vi "Reason List.vi"(8 "error in (no error)":errorcluster, 11 "Ref In":T1={"MS SQL Connection"=refnum, "UDL File"=path "", "Time"="", "DCODE"="", "WIP+1"=0, "MC No?"=0, "POKAYOKE?"=FALSE, "Expected Result"="", "Result [Status]"="", "Clock"=0.0, "RFID"="", "WIP Queue"=refnum, "TS Parameter"={"ProfitCenterCode"="", "LineCode"="", "WorkOrderNumber"="", "Model"="", "Model_with_Prefix"="", "VendorCode"="", "SetParameterDateCode"="", "PokaYoke"=0, "Target"=1, "Live_DateCode"="", "CustomerPartNumber"="", "Hand"="", "sBarcode"=FALSE, "FCA"=0, "Ent_Stamp"=timestamp(0 s since 1904-01-01), "STS_CD"=0.0}, "Data_Queue"=[], "RFID Serial No."=""} {"TS Parameter"."FCA" format="%01d"; "TS Parameter"."Target" min=1 max=100000; "TS Parameter"."PokaYoke" min=0 max=1}) -> (0 "error out":errorcluster)   [LabVIEW 2020]
uses:
  Controls/Loss_type.ctl
  Controls/TD SQL.ctl
  <vilib>/addons/database/Connection.llb/Conn ObjectReference.ctl
  Controls/WIP_State.ctl
  Controls/TS_Parameter.ctl
  <vilib>/addons/database/NI_Database_API.lvlib
panel:
  in  "Refresh":bool
  in  "Exit":bool
  in  "Del":bool
  in  "Change":bool
  in  "Add":bool
  in  "Reason":string
  in  "Code":i32(listbox)
  in  "Code Type":T4
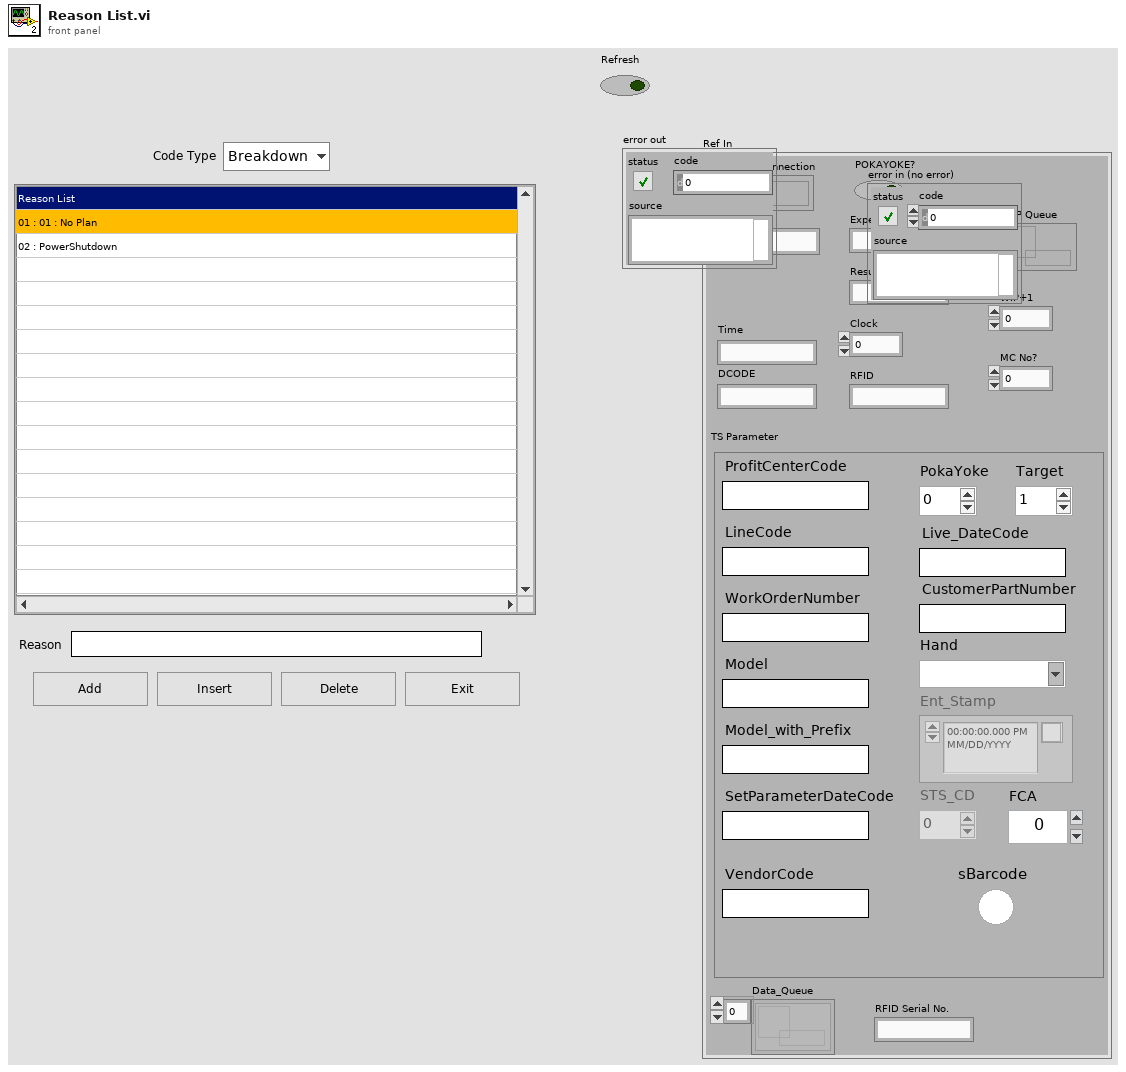
[diagram p1: front panel]
types:
  T1 = typedef "TD SQL.ctl" = cluster{"MS SQL Connection":T2, "UDL File":path, "Time":string, "DCODE":string, "WIP+1":i64, "MC No?":i32, "POKAYOKE?":bool, "Expected Result":string, "Result [Status]":string, "Clock":dbl, "RFID":string, "WIP Queue":refnum<queue>, "TS Parameter":T3, "Data_Queue":refnum<queue>[], "RFID Serial No.":string}
  T2 = typedef "NI_Database_API.lvlib/Conn ObjectReference.ctl" = refnum<k1>
  T3 = typedef "TS_Parameter.ctl" = cluster{"ProfitCenterCode":string, "LineCode":string, "WorkOrderNumber":string, "Model":string, "Model_with_Prefix":string, "VendorCode":string, "SetParameterDateCode":string, "PokaYoke":i32, "Target":i32, "Live_DateCode":string, "CustomerPartNumber":string, "Hand":string, "sBarcode":bool, "FCA":i32, "Ent_Stamp":timestamp, "STS_CD":dbl}
  T4 = typedef "Loss_type.ctl" = enum16{"Breakdown", "Bookout"}
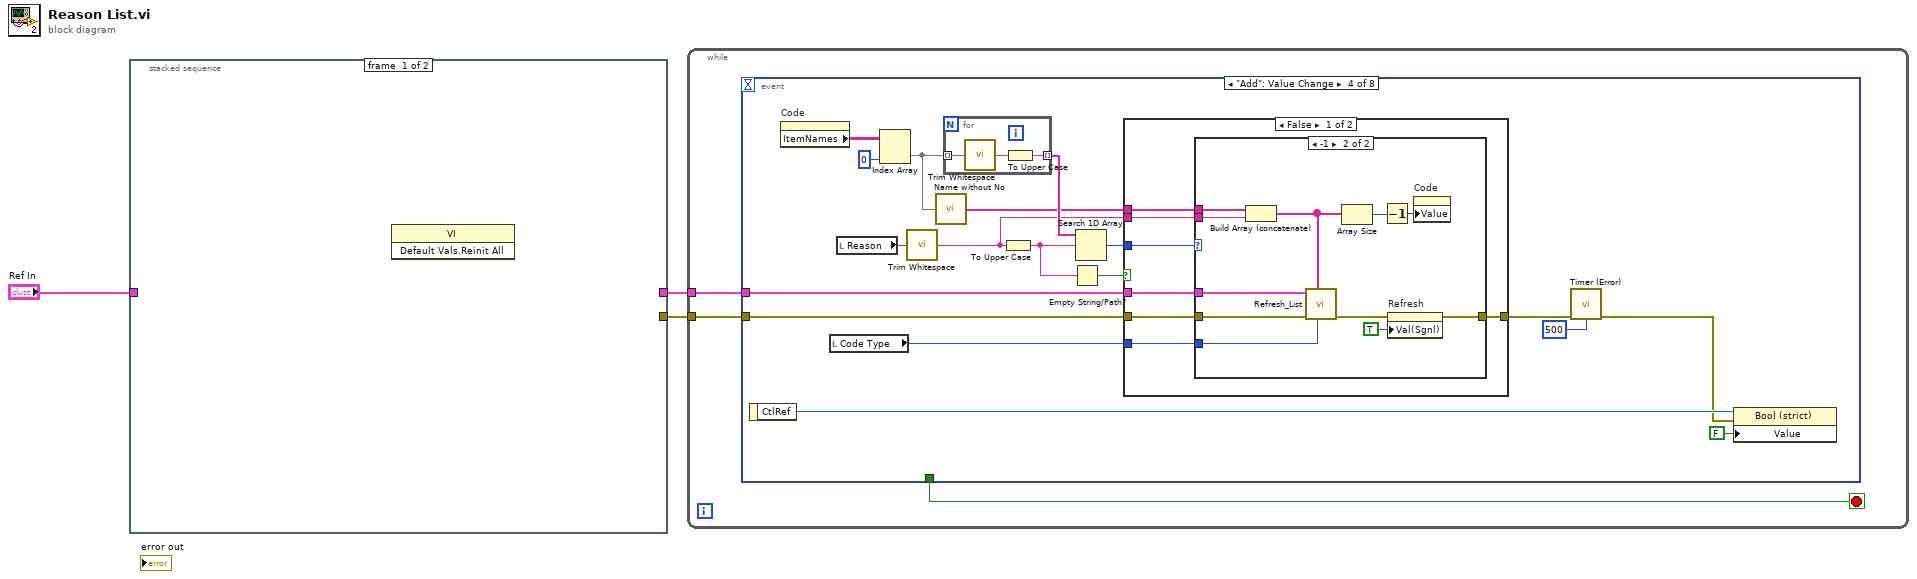
[diagram p0: block diagram]
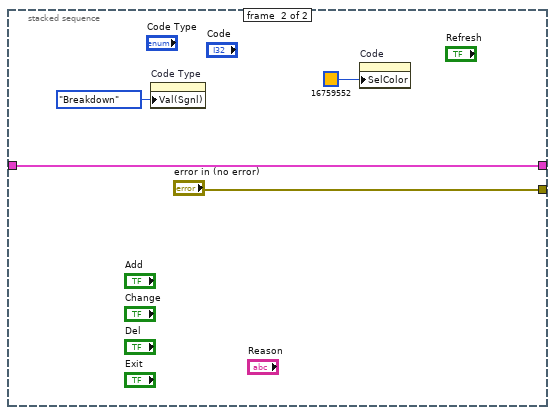
[diagram p2: hidden frame]
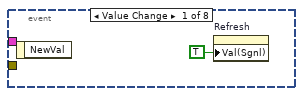
[diagram p3: hidden frame]
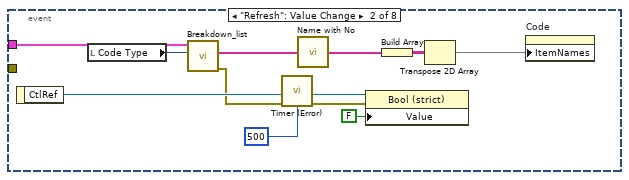
[diagram p4: hidden frame]
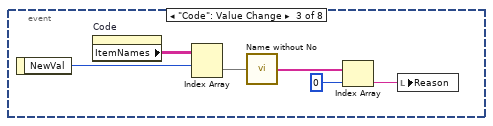
[diagram p5: hidden frame]
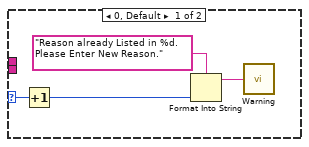
[diagram p6: hidden frame]
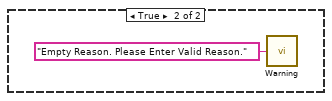
[diagram p7: hidden frame]
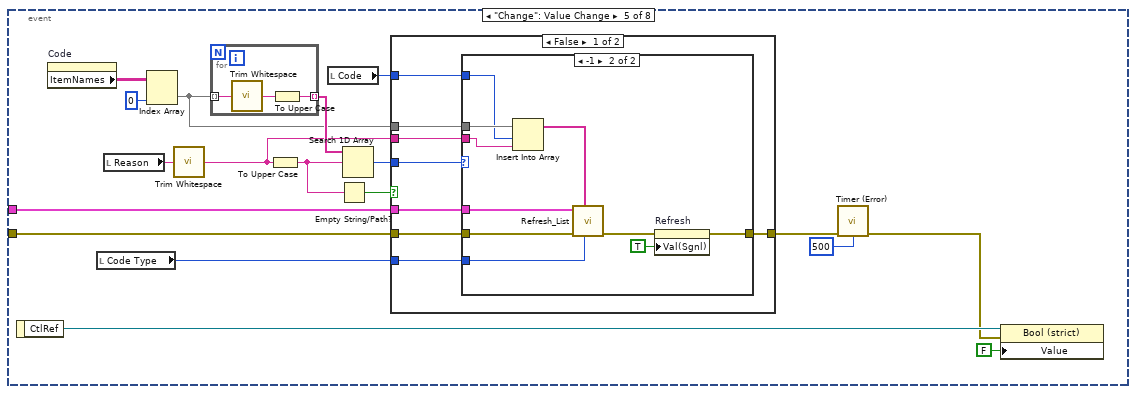
[diagram p8: hidden frame]
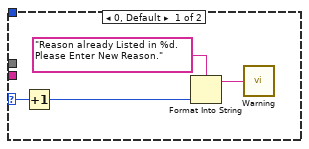
[diagram p9: hidden frame]
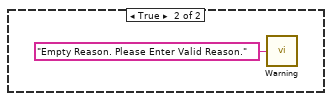
[diagram p10: hidden frame]
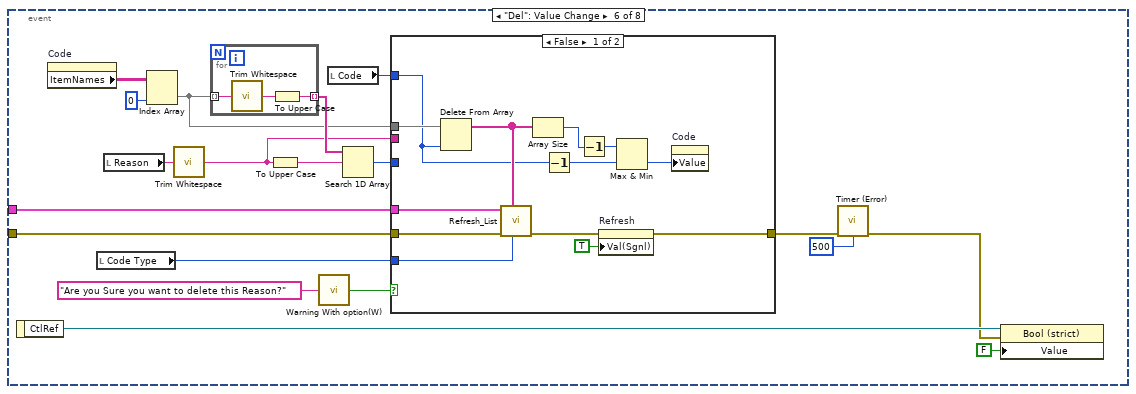
[diagram p11: hidden frame]
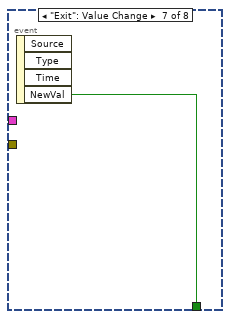
[diagram p13: hidden frame]
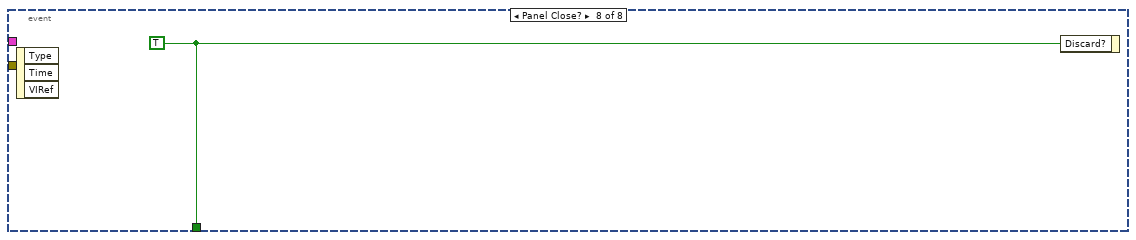
[diagram p14: hidden frame]
diagram:
  n1 = stacked-sequence {
    tunnel: [_ w4] -> w3
    tunnel: [_ "error in (no error)"] -> w2
    tunnel: "Ref In" -> [_ w4]
    frame #0 {
      n2 = invoke class="VI" method="Default Vals.Reinit All"() -> ()  [unwired: 3 in, 3 out]
    }
    frame #1 {
      n3 = property on="Code Type" class="Enum (strict)"("Val(Sgnl)"=Loss_type."Breakdown" ("Value (Signaling)")) -> ()  [unwired: 2 in, 2 out]
      n4 = property on="Code" class="MCListbox (strict)"("SelColor"=u32 16759552 ("Selection Color")) -> ()  [unwired: 2 in, 2 out]
    }
  }
  n5 = while {
    tunnel: w3 -> [w9]
    tunnel: w2 -> [w8]
    stop <- w10 stop-if-true
    n6 = event shown="[3] \"Add\": Value Change" {
      selector: _ -> [_ _ _ _ _ _ _ _]
      dyn-events: _ -> [_ _ _ _ _ _ _ _]
      timeout: _ -> [_ _ _ _ _ _ _ _]
      tunnel: [_ _ _ _ _ _ w152 w153] -> w10
      tunnel: w9 -> [_ w22 _ w35 w79 w125 _ _]
      tunnel: w8 -> [_ _ _ w42 w86 w131 _ _]
      event Value Change {
        n7 = event-data() -> ()  [unwired: 1 in, 1 out]
        n8 = property on="Refresh" class="Bool (strict)"("Val(Sgnl)"=TRUE ("Value (Signaling)")) -> ()  [unwired: 2 in, 2 out]
      }
      event "Refresh": Value Change {
        n9 = event-data() -> ("CtlRef"=w20:refnum<vi>)  [unwired: 1 in]
        n10 = local read "Code Type"() -> (w21:T4)
        n11 = call "Breakdown_list.vi"("Reason Type"=w21, "Ref In"=w22) -> ("error out"=w18:errorcluster, "Reason List"=w13:string[])  [unwired: 6 in, 2 out]
        n12 = call <userlib>:"Timer (Error).vi"("error in (no error)"=w18, "milliseconds to wait"=u32 500) -> ("error out"=w17:errorcluster)  [unwired: 13 in]
        n13 = call <userlib>:"Name with No.vi"("Seq Name In"=w13) -> ("Seq Name (No.)"=w12:string[])  [unwired: 14 in]
        n14 = property class="Bool (strict)"(reference=w20, error in=w17, "Value"=FALSE ("Value (Signaling)")) -> ()  [unwired: 2 out]
        n15 = Build Array(w12) -> (w15:string[][])
        n16 = Transpose 2D Array(2D array=w15) -> (transposed array=w14:string[][])
        n17 = property on="Code" class="MCListbox (strict)"("ItemNames"=w14) -> ()  [unwired: 2 in, 2 out]
      }
      event "Code": Value Change {
        n18 = event-data() -> ("NewVal"=w27:i32)  [unwired: 1 in]
        n19 = property on="Code" class="MCListbox (strict)"() -> ("ItemNames"=w28:string[][])  [unwired: 2 in, 2 out]
        n20 = Index Array(array=w28, index (row)=w27) -> (element=w26:string[])  [unwired: 1 in]
        n21 = call <userlib>:"Name without No.vi"("Seq Name (No.)"=w26) -> ("Seq Name Out"=w25:string[])  [unwired: 14 in]
        n22 = Index Array(array=w25, index=0 ("disabled index (col)")) -> (element=w23:string)
        n23 = local write "Reason"(w23) -> ()
      }
      event "Add": Value Change {
        n24 = event-data() -> ("CtlRef"=w41:refnum<vi>)  [unwired: 1 in]
        n25 = property on="Code" class="MCListbox (strict)"() -> ("ItemNames"=w46:string[][])  [unwired: 2 in, 2 out]
        n26 = local read "Code Type"() -> (w34:T4)
        n27 = local read "Reason"() -> (w36:string)
        n28 = Index Array(array=w46, index (col)=0 ("disabled index (col)")) -> (element=w37:string[])  [unwired: 1 in]
        n29 = call <vilib>:"Trim Whitespace.vi"("string"=w36) -> ("trimmed string"=w33:string)  [unwired: 1 in]
        n30 = call <userlib>:"Name without No.vi"("Seq Name (No.)"=w37) -> ("Seq Name Out"=w29:string[])  [unwired: 14 in]
        n31 = for {
          tunnel: w37 -> [w72] mode=indexing
          tunnel: [w70] -> w44 mode=indexing
          n32 = call <vilib>:"Trim Whitespace.vi"("string"=w72) -> ("trimmed string"=w71:string)  [unwired: 1 in]
          n33 = To Upper Case(1:w71) -> (0:w70:string)
        }
        n34 = To Upper Case(1:w33) -> (0:w39:string)
        n35 = Empty String/Path?(string/path=w39) -> (empty?=w38:bool)
        n36 = Search 1D Array(1D array=w44, element=w39) -> (index of element=w43:i32)  [unwired: 1 in]
        n37 = case shown="False" w38 {
          tunnel: w43 -> [w47 _]
          tunnel: w42 -> [w53 _]
          tunnel: [w52 _] -> w32
          tunnel: w29 -> [w51 _]
          tunnel: w33 -> [w50 _]
          tunnel: w35 -> [w49 _]
          tunnel: w34 -> [w48 _]
          frame False {
            n38 = case shown="-1" w47 {
              selector: w47 -> [w57 _]
              tunnel: [_ w61] -> w52
              tunnel: w53 -> [_ w66]
              tunnel: w51 -> [_ w68]
              tunnel: w50 -> [_ w67]
              tunnel: w49 -> [_ w65]
              tunnel: w48 -> [_ w64]
              frame 0, Default {
                n39 = Increment(x=w57) -> (x+1=w54:i32)
                n40 = Format Into String(format string="Reason already Listed in %d. Please Enter New Reason." ("Warning in"), w54) -> (resulting string=w55:string)  [unwired: 2 in, 1 out]
                n41 = call <userlib>:"Warning .vi"("Warning in"=w55) -> ()  [unwired: 15 in]
              }
              frame -1 {
                n42 = Build Array (concatenate)(w68, w67) -> (w60:string[])
                n43 = call "Refresh_List.vi"("Code Type"=w64, "List"=w60, "error in (no error)"=w66, "Ref In"=w65) -> ("error out"=w62:errorcluster)  [unwired: 7 in]
                n44 = Array Size(array=w60) -> (size(s)=w59:i32)
                n45 = Decrement(x=w59) -> (x-1=w58:i32)
                n46 = property on="Refresh" class="Bool (strict)"(error in=w62, "Val(Sgnl)"=TRUE ("Value (Signaling)")) -> (error out=w61:errorcluster)  [unwired: 1 in, 1 out]
                n47 = property on="Code" class="MCListbox (strict)"("Value"=w58) -> ()  [unwired: 2 in, 2 out]
              }
            }
          }
          frame True {
            n48 = call <userlib>:"Warning .vi"("Warning in"="Empty Reason. Please Enter Valid Reason.") -> ()  [unwired: 15 in]
          }
        }
        n49 = call <userlib>:"Timer (Error).vi"("error in (no error)"=w32, "milliseconds to wait"=u32 500) -> ("error out"=w31:errorcluster)  [unwired: 13 in]
        n50 = property class="Bool (strict)"(reference=w41, error in=w31, "Value"=FALSE) -> ()  [unwired: 2 out]
      }
      event "Change": Value Change {
        n51 = event-data() -> ("CtlRef"=w85:refnum<vi>)  [unwired: 1 in]
        n52 = property on="Code" class="MCListbox (strict)"() -> ("ItemNames"=w90:string[][])  [unwired: 2 in, 2 out]
        n53 = local read "Code Type"() -> (w78:T4)
        n54 = local read "Reason"() -> (w80:string)
        n55 = Index Array(array=w90, index (col)=0 ("disabled index (col)")) -> (element=w81:string[])  [unwired: 1 in]
        n56 = call <vilib>:"Trim Whitespace.vi"("string"=w80) -> ("trimmed string"=w77:string)  [unwired: 1 in]
        n57 = for {
          tunnel: w81 -> [w116] mode=indexing
          tunnel: [w114] -> w88 mode=indexing
          n58 = call <vilib>:"Trim Whitespace.vi"("string"=w116) -> ("trimmed string"=w115:string)  [unwired: 1 in]
          n59 = To Upper Case(1:w115) -> (0:w114:string)
        }
        n60 = To Upper Case(1:w77) -> (0:w83:string)
        n61 = local read "Code"() -> (w73:i32)
        n62 = Empty String/Path?(string/path=w83) -> (empty?=w82:bool)
        n63 = Search 1D Array(1D array=w88, element=w83) -> (index of element=w87:i32)  [unwired: 1 in]
        n64 = case shown="False" w82 {
          tunnel: w87 -> [w92 _]
          tunnel: w86 -> [w98 _]
          tunnel: [w97 _] -> w76
          tunnel: w81 -> [w96 _]
          tunnel: w77 -> [w95 _]
          tunnel: w79 -> [w94 _]
          tunnel: w78 -> [w93 _]
          tunnel: w73 -> [w91 _]
          frame False {
            n65 = case shown="-1" w92 {
              selector: w92 -> [w102 _]
              tunnel: [_ w105] -> w97
              tunnel: w98 -> [_ w111]
              tunnel: w96 -> [_ w112]
              tunnel: w95 -> [_ w104]
              tunnel: w94 -> [_ w109]
              tunnel: w93 -> [_ w108]
              tunnel: w91 -> [_ w103]
              frame 0, Default {
                n66 = Increment(x=w102) -> (x+1=w99:i32)
                n67 = Format Into String(format string="Reason already Listed in %d. Please Enter New Reason." ("Warning in"), w99) -> (resulting string=w100:string)  [unwired: 2 in, 1 out]
                n68 = call <userlib>:"Warning .vi"("Warning in"=w100) -> ()  [unwired: 15 in]
              }
              frame -1 {
                n69 = Insert Into Array(array=w112, index=w103, new element=w104) -> (w110:string[])
                n70 = call "Refresh_List.vi"("Code Type"=w108, "List"=w110, "error in (no error)"=w111, "Ref In"=w109) -> ("error out"=w106:errorcluster)  [unwired: 7 in]
                n71 = property on="Refresh" class="Bool (strict)"(error in=w106, "Val(Sgnl)"=TRUE ("Value (Signaling)")) -> (error out=w105:errorcluster)  [unwired: 1 in, 1 out]
              }
            }
          }
          frame True {
            n72 = call <userlib>:"Warning .vi"("Warning in"="Empty Reason. Please Enter Valid Reason.") -> ()  [unwired: 15 in]
          }
        }
        n73 = call <userlib>:"Timer (Error).vi"("error in (no error)"=w76, "milliseconds to wait"=u32 500) -> ("error out"=w75:errorcluster)  [unwired: 13 in]
        n74 = property class="Bool (strict)"(reference=w85, error in=w75, "Value"=FALSE) -> ()  [unwired: 2 out]
      }
      event "Del": Value Change {
        n75 = event-data() -> ("CtlRef"=w130:refnum<vi>)  [unwired: 1 in]
        n76 = property on="Code" class="MCListbox (strict)"() -> ("ItemNames"=w135:string[][])  [unwired: 2 in, 2 out]
        n77 = local read "Code Type"() -> (w124:T4)
        n78 = local read "Reason"() -> (w126:string)
        n79 = Index Array(array=w135, index (col)=0 ("disabled index (col)")) -> (element=w127:string[])  [unwired: 1 in]
        n80 = call <vilib>:"Trim Whitespace.vi"("string"=w126) -> ("trimmed string"=w123:string)  [unwired: 1 in]
        n81 = for {
          tunnel: w127 -> [w151] mode=indexing
          tunnel: [w149] -> w133 mode=indexing
          n82 = call <vilib>:"Trim Whitespace.vi"("string"=w151) -> ("trimmed string"=w150:string)  [unwired: 1 in]
          n83 = To Upper Case(1:w150) -> (0:w149:string)
        }
        n84 = To Upper Case(1:w123) -> (0:w128:string)
        n85 = call <userlib>:"Warning With option(W).vi"("Warning in"="Are you Sure you want to delete this Reason?") -> ("Cancel ?"=w117:bool)  [unwired: 13 in, 1 out]
        n86 = local read "Code"() -> (w119:i32)
        n87 = Search 1D Array(1D array=w133, element=w128) -> (index of element=w132:i32)  [unwired: 1 in]
        n88 = case shown="False" w117 {
          tunnel: w132 -> [_ _]
          tunnel: w131 -> [w148 _]
          tunnel: [w147 _] -> w122
          tunnel: w127 -> [w146 _]
          tunnel: w123 -> [_ _]
          tunnel: w125 -> [w145 _]
          tunnel: w124 -> [w144 _]
          tunnel: w119 -> [w139 _]
          frame False {
            n89 = Delete From Array(array=w146, index=w139) -> (array with subset deleted=w141:string[])  [unwired: 1 in, 1 out]
            n90 = call "Refresh_List.vi"("Code Type"=w144, "List"=w141, "error in (no error)"=w148, "Ref In"=w145) -> ("error out"=w142:errorcluster)  [unwired: 7 in]
            n91 = Array Size(array=w141) -> (size(s)=w140:i32)
            n92 = Decrement(x=w139) -> (x-1=w136:i32)
            n93 = Decrement(x=w140) -> (x-1=w137:i32)
            n94 = property on="Refresh" class="Bool (strict)"(error in=w142, "Val(Sgnl)"=TRUE ("Value (Signaling)")) -> (error out=w147:errorcluster)  [unwired: 1 in, 1 out]
            n95 = Max & Min(x=w137, y=w136) -> (min(x,y)=w138:i32)  [unwired: 1 out]
            n96 = property on="Code" class="MCListbox (strict)"("Value"=w138) -> ()  [unwired: 2 in, 2 out]
          }
          frame True {
          }
        }
        n97 = call <userlib>:"Timer (Error).vi"("error in (no error)"=w122, "milliseconds to wait"=u32 500) -> ("error out"=w121:errorcluster)  [unwired: 13 in]
        n98 = property class="Bool (strict)"(reference=w130, error in=w121, "Value"=FALSE) -> ()  [unwired: 2 out]
      }
      event "Exit": Value Change {
        n99 = event-data() -> ("NewVal"=w152:bool)  [unwired: 1 in, 3 out]
      }
      event Panel Close? {
        w153 = TRUE ("Discard?")
        n100 = event-data() -> ()  [unwired: 1 in, 3 out]
        n101 = event-data("Discard?"=w153) -> ()  [unwired: 1 in, 1 out]
      }
    }
  }
